vi "GlobalVariable.vi"() -> ()   [LabVIEW 2013]
panel:
  in  "列累计":string[](array[string])
  in  "次数":u32
  in  "周期":u32
  in  "计数清零":bool
  out "Success":bool
  out "Exit":bool
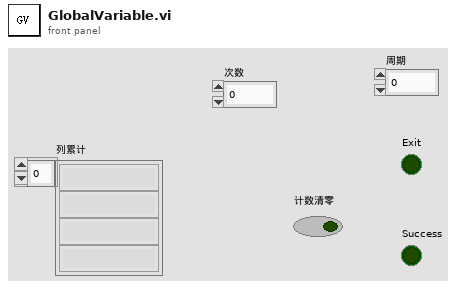
[diagram p1: front panel]
diagram:
